vi "IMAQ_Attribute2Control_Str.vi"(3 "error in (no error)":errorcluster, 4 "IMAQ Attribute":variant, 5 "Refnum (String)":refnum<vi>) -> (0 "error out":errorcluster, 1 "dup IMAQ Attribute":variant)   [LabVIEW 2012, in "HGF_VisionTools.lvlib"]
doc: "This Polymorphic VI set IMAQ control properties of type string according to variant inputp value and its attribute."
uses:
  HGF_VisionTools.lvlib
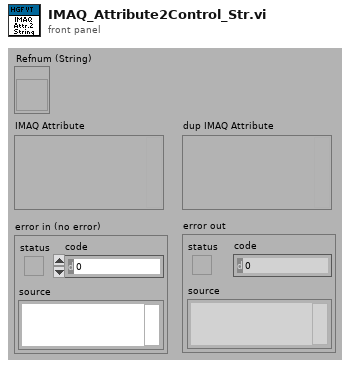
[diagram p1: front panel]
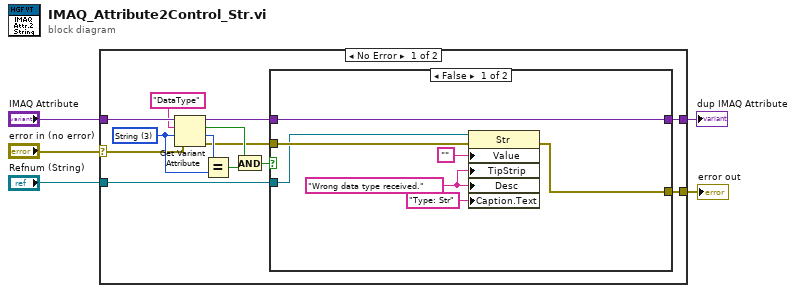
[diagram p0: block diagram]
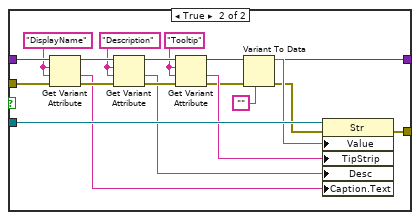
[diagram p2: hidden frame]
diagram:
  n1 = case shown="No Error" "error in (no error)" {
    selector: "error in (no error)" -> [w11 w46]
    tunnel: "IMAQ Attribute" -> [w18 w45]
    tunnel: "Refnum (String)" -> [w8 _]
    tunnel: [w7 w46] -> w2
    tunnel: [w6 w45] -> w1
    frame No Error {
      w15 = u32 3 items=["U32", "I64", "DBL", "String", "Enum", "Bool", "Command"] ("Type")
      n2 = Get Variant Attribute(Variant=w18, name="DataType", default value (empty Variant)=w15, error in=w11) -> (duplicate Variant=w10:variant, found=w14:bool, value=w16:u32, error out=w9:errorcluster)
      n3 = Equal?(x=w16, y=w15) -> (x = y?=w13:bool)
      n4 = And(x=w14, y=w13) -> (x .and. y?=w12:bool)
      n5 = case shown="False" w12 {
        tunnel: w10 -> [w25 w44]
        tunnel: w9 -> [w23 w43]
        tunnel: w8 -> [w22 w42]
        tunnel: [w21 w28] -> w7
        tunnel: [w25 w27] -> w6
        frame False {
          w24 = "Wrong data type received." ("Tip Strip")
          n6 = property class="Str"(reference=w22, error in=w23, "Value"="", "TipStrip"=w24, "Desc"=w24, "Caption.Text"="Type: Str") -> (error out=w21:errorcluster)  [unwired: 1 out]
        }
        frame True {
          w33 = "Tooltip" ("name")
          w32 = "Description" ("name")
          w31 = "DisplayName" ("name")
          n7 = Get Variant Attribute(Variant=w44, name=w31, default value (empty Variant)=w31, error in=w43) -> (duplicate Variant=w39:variant, value=w29:string, error out=w40:errorcluster)  [unwired: 1 out]
          n8 = Get Variant Attribute(Variant=w39, name=w32, default value (empty Variant)=w32, error in=w40) -> (duplicate Variant=w38:variant, value=w30:string, error out=w41:errorcluster)  [unwired: 1 out]
          n9 = Get Variant Attribute(Variant=w38, name=w33, default value (empty Variant)=w33, error in=w41) -> (duplicate Variant=w27:variant, value=w34:string, error out=w26:errorcluster)  [unwired: 1 out]
          n10 = Variant To Data(error in=w26, type="" ("Value"), Variant=w27) -> (data=w37:string, error out=w36:errorcluster)
          n11 = property class="Str"(reference=w42, error in=w36, "Value"=w37, "TipStrip"=w34, "Desc"=w30, "Caption.Text"=w29) -> (error out=w28:errorcluster)  [unwired: 1 out]
        }
      }
    }
    frame Error {
    }
  }
  "error out" <- w2
  "dup IMAQ Attribute" <- w1
